vi "PhaseRef.vi"(9 "phase per sample (rad)":dbl=1e-06 format="%#_13g", 10 "phase reference channel":i32, 11 "Phase in":dbl[][](array[numeric])) -> (3 "Phase ref":dbl[](array[numeric]))   [LabVIEW 2018]
uses:
  controls/Channel_select_2fpga.ctl
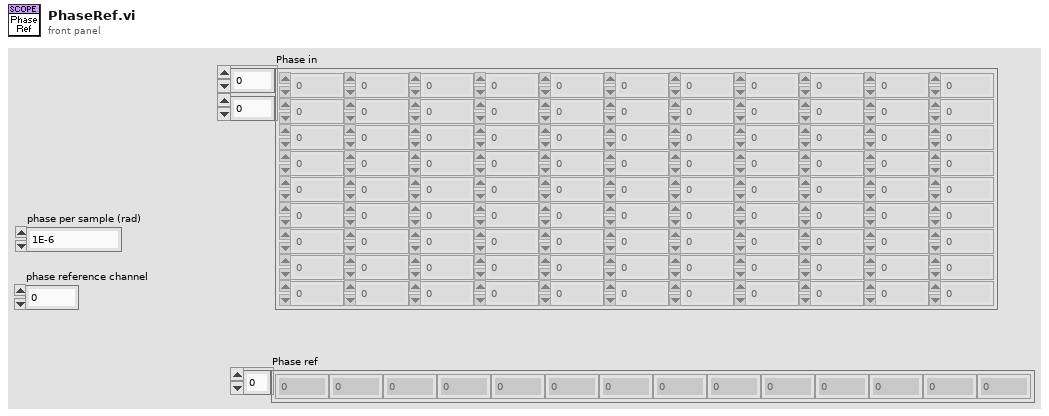
[diagram p1: front panel]
types:
  T1 = typedef "Channel_select_2fpga.ctl" = enum16{"5785 - Ch0", "5785 - Ch1 cavity", "5785 - Ch1", "5761 - Ch0", "5761 - Ch1", "5761 - Ch2", "5761 - Ch3", "Fixed"}
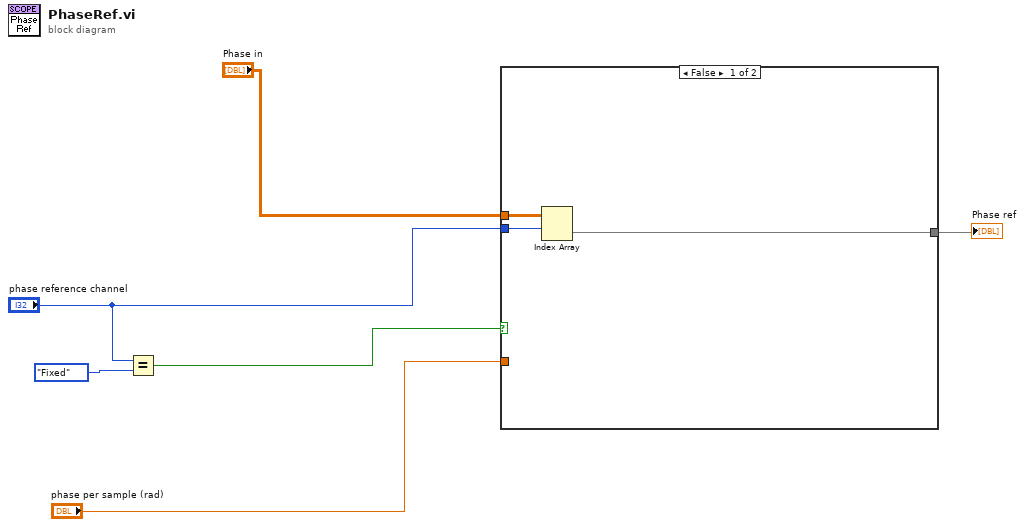
[diagram p0: block diagram]
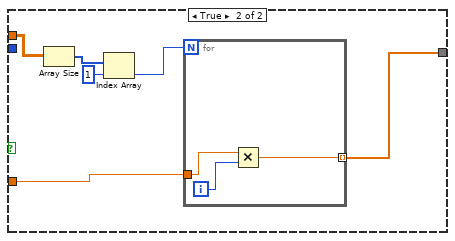
[diagram p2: hidden frame]
diagram:
  n1 = Equal?(x="phase reference channel", y=Channel_select_2fpga."Fixed" ("Reference for phase")) -> (x = y?=w3:bool)
  n2 = case shown="False" w3 {
    tunnel: [w9 w10] -> w6
    tunnel: "phase reference channel" -> [w8 _]
    tunnel: "Phase in" -> [w7 w15]
    tunnel: "phase per sample (rad)" -> [_ w11]
    frame False {
      n3 = Index Array(array=w7, index (row)=w8) -> (element=w9:dbl[])  [unwired: 1 in]
    }
    frame True {
      n4 = Array Size(array=w15) -> (size(s)=w14:i32[])
      n5 = Index Array(array=w14, index=1) -> (element=w13:i32)
      n6 = for {
        N: w13 -> [_]
        tunnel: w11 -> [w17]
        tunnel: [w16] -> w10 mode=indexing
        i -> [w18]
        n7 = Multiply(x=w17, y=w18) -> (x*y=w16:dbl)
      }
    }
  }
  "Phase ref" <- w6
